vi "Auton PickUpRC.vi"() -> ()   [LabVIEW 2014]
uses:
  Robot Global Data.vi
panel:
  out "Waveform Chart":dbl(graph)
  in  "Wait Time between each step":dbl=0.5
  out "Current Step 2":string
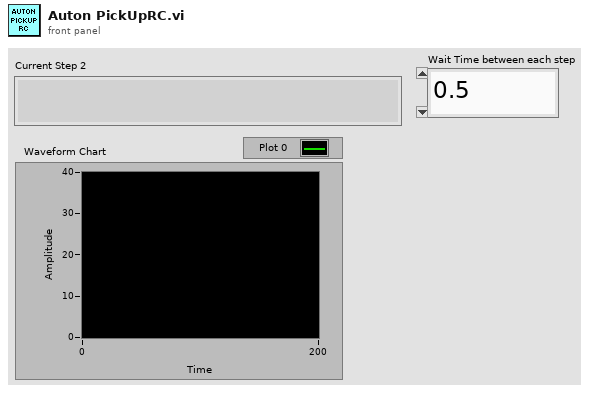
[diagram p1: front panel]
types:
  T1 = typedef "WPI_EncoderDevRef.ctl" = cluster{"DevStatus":errorcluster, "EncoderIndex":T2, "CounterIndex":T3, "DistancePerCount":dbl, "Decoding Type":T4}
  T2 = typedef "FPGA_EncoderIdx.ctl" = enum8{"Enc 0", "Enc 1", "Enc 2", "Enc 3", "Enc 4", "Enc 5", "Enc 6", "Enc 7", "Invalid"}
  T3 = typedef "FPGA_CounterCtrSystemIndex.ctl" = enum8{"Ctr 0", "Ctr 1", "Ctr 2", "Ctr 3", "Ctr 4", "Ctr 5", "Ctr 6", "Ctr 7", "Invalid"}
  T4 = typedef "WPI_EncoderType.ctl" = enum16{"1x", "2x", "4x"}
  T5 = typedef "WPI_MotorControlDeviceRef.ctl" = cluster{"DeviceStatus":errorcluster, "Type":T6, "PWM":cluster{"Controller":T7, "PWM Channel":T8, "DeadBand":T9}, "CAN":cluster{"Device Number":u8, "Control Mode":T10, "Semaphore":T11, "Max Vout":dbl, "TalonSRX Control Mode":T12}, "Invert":bool, "TransformRef":T13, "InvTransformRef":T13}
  T6 = typedef "WPI_MotorControlType.ctl" = enum16{"PWM", "CAN", "CANTalonSRX"}
  T7 = typedef "FPGA_TypedefDigitalModule.ctl" = enum16{"Controller 1"}
  T8 = typedef "FPGA_DIOPWMChannel.ctl" = enum8{"PWM 0", "PWM 1", "PWM 2", "PWM 3", "PWM 4", "PWM 5", "PWM 6", "PWM 7", "PWM 8", "PWM 9", "PWM MXP 0", "PWM MXP 1", "PWM MXP 2", "PWM MXP 3", "PWM MXP 4", "PWM MXP 5", "PWM MXP 6", "PWM MXP 7", "PWM MXP 8", "PWM MXP 9", "Invalid"}
  T9 = typedef "WPI_PWMDeadband.ctl" = cluster{"Name":string, "maxPositivePwm":i32, "minPositivePwm":i32, "centerPwm":i32, "maxNegativePwm":i32, "minNegativePwm":i32, "angularRange":u16}
  T10 = typedef "WPI_CANJaguar_ControlMode.ctl" = enum8{"Percent VBus", "Current", "Speed", "Position", "Voltage"}
  T11 = typedef "Semaphore RefNum" = refnum<k1>
  T12 = typedef "WPI_CANTalonSRX_APIControlMode.ctl" = enum8{"Percent VBus", "Speed", "Position", "Slave", "Unchanged / Invalid"}
  T13 = typedef "WPI_PWMTransform_ConPane.ctl" = refnum<vi>
  T14 = enum16{"Claw State Opening", "Claw State Opened"}
  T15 = enum16{"Claw State Open", "Claw State Closed", "Claw State Do Nothing"}
  T16 = enum16{"Elevator State Bottom", "Elevator State Clear a Tote", "Elevator State Carry a  RC", "Elevator do Nothing"}
  T17 = enum16{"Elevator Heading to Bottom", "Elevator Reached Bottom"}
  T18 = enum16{"Claw State Closing", "Claw State Closed"}
  T19 = enum16{"Claw State Closing", "Claw State Closed", "Squeeze"}
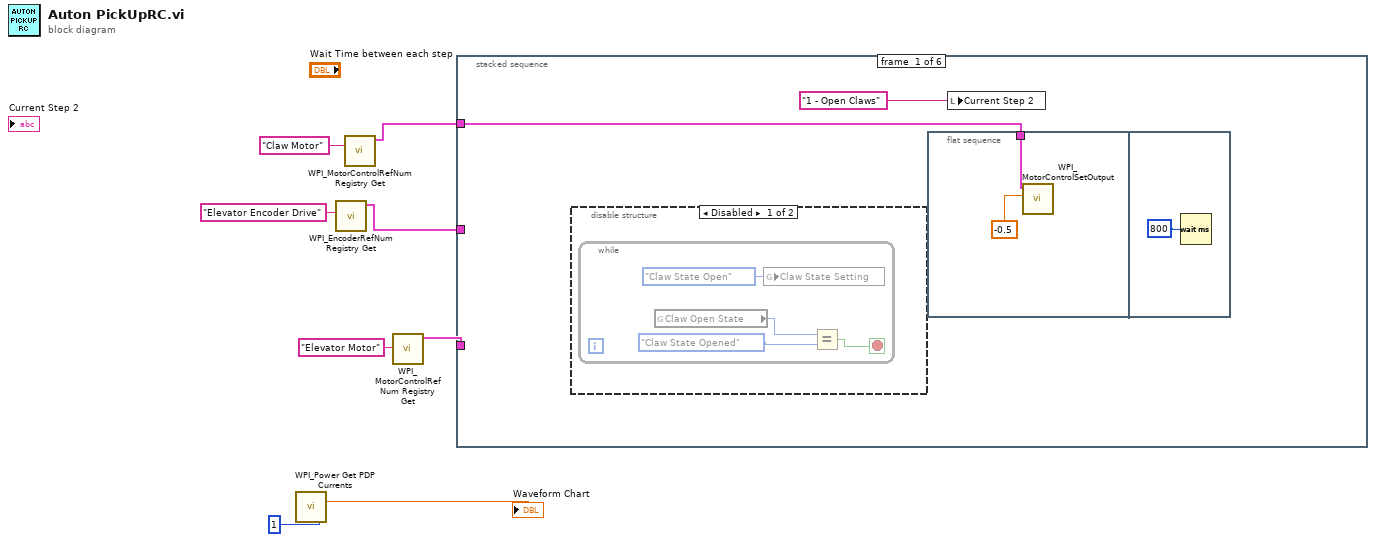
[diagram p0: block diagram]
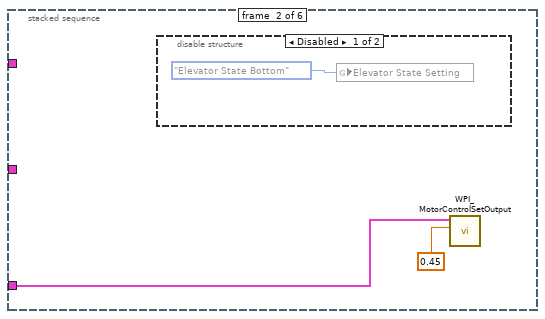
[diagram p3: hidden frame]
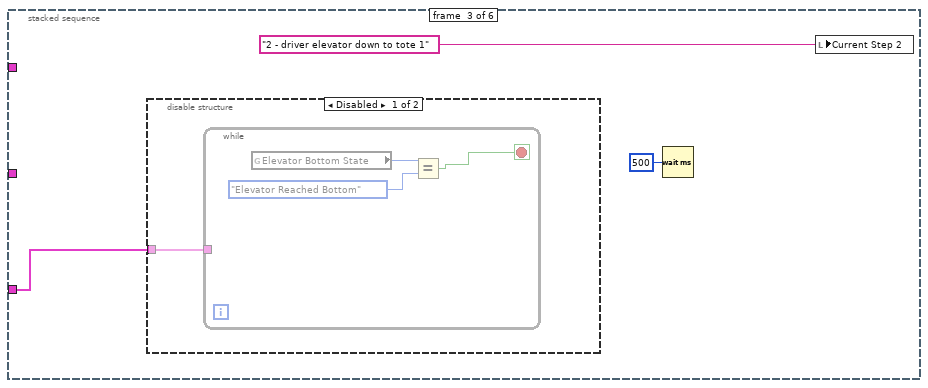
[diagram p5: hidden frame]
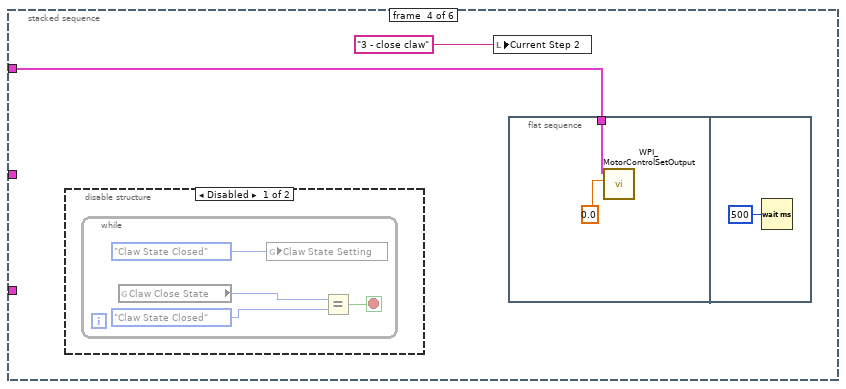
[diagram p7: hidden frame]
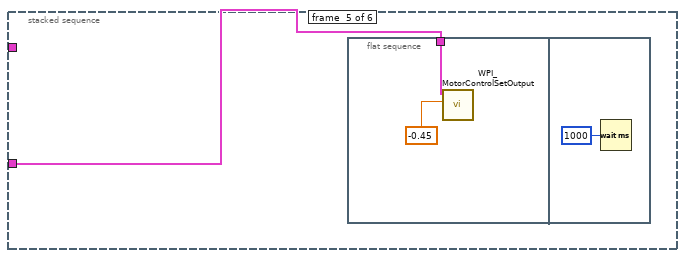
[diagram p9: hidden frame]
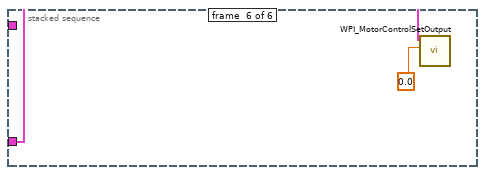
[diagram p10: hidden frame]
diagram:
  n1 = call <vilib>:"WPI_Power Get PDP Currents.vi"("PDP Channel"=1) -> ("current (A)"=→"Waveform Chart":dbl)  [unwired: 12 in, 2 out]
  n2 = call <vilib>:"WPI_EncoderRefNum Registry Get.vi"("refnum name"="Elevator Encoder Drive") -> ("EncoderDevRef"=w5:T1)  [unwired: 9 in, 1 out]
  n3 = call <vilib>:"WPI_MotorControlRefNum Registry Get.vi"("refnum name"="Claw Motor") -> ("MotorControlDevRef"=w1:T5)  [unwired: 9 in, 1 out]
  n4 = call <vilib>:"WPI_MotorControlRefNum Registry Get.vi"("refnum name"="Elevator Motor") -> ("MotorControlDevRef"=w7:T5)  [unwired: 9 in, 1 out]
  n5 = stacked-sequence {
    tunnel: w7 -> [_ w19 w22 _ w37 w42]
    tunnel: w5 -> [_ _ _ _ _ _]
    tunnel: w1 -> [w9 _ _ w28 _ _]
    frame #0 {
      n6 = disable-structure shown="Disabled" {
        frame Disabled {
          n7 = while {
            stop <- w15 stop-if-true
            n8 = global read "Robot Global Data.vi" "Claw Open State"() -> (w16:T14)
            n9 = global write "Robot Global Data.vi" "Claw State Setting"(T15."Claw State Open" ("Enum")) -> ()
            n10 = Equal?(x=w16, y=T14."Claw State Opened" ("Claw Open State")) -> (x = y?=w15:bool)
          }
        }
        frame Enabled {
        }
      }
      n11 = flat-sequence {
        tunnel: w9 -> [w11]
        frame #0 {
          n12 = call <vilib>:"WPI_MotorControlSetOutput.vi"("Output"=-0.5, "MotorControlDevRef"=w11) -> ()  [unwired: 7 in, 3 out]
        }
        frame #1 {
          n13 = Wait (ms)(milliseconds to wait=u32 800) -> ()  [unwired: 1 out]
        }
      }
      n14 = local write "Current Step 2"("1 - Open Claws" ("Current Step")) -> ()
    }
    frame #1 {
      n15 = disable-structure shown="Disabled" {
        frame Disabled {
          n16 = global write "Robot Global Data.vi" "Elevator State Setting"(T16."Elevator State Bottom" ("Elevator State Setting")) -> ()
        }
        frame Enabled {
        }
      }
      n17 = call <vilib>:"WPI_MotorControlSetOutput.vi"("Output"=0.45, "MotorControlDevRef"=w19) -> ()  [unwired: 7 in, 3 out]
    }
    frame #2 {
      n18 = disable-structure shown="Disabled" {
        disable-tunnel: w22 -> [w24 _]
        frame Disabled {
          n19 = while {
            tunnel: w24 -> [_]
            stop <- w25 stop-if-true
            n20 = global read "Robot Global Data.vi" "Elevator Bottom State"() -> (w27:T17)
            n21 = Equal?(x=w27, y=T17."Elevator Reached Bottom" ("Elevator Bottom State")) -> (x = y?=w25:bool)
          }
        }
        frame Enabled {
        }
      }
      n22 = Wait (ms)(milliseconds to wait=u32 500) -> ()  [unwired: 1 out]
      n23 = local write "Current Step 2"("2 - driver elevator down to tote 1" ("Current Step")) -> ()
    }
    frame #3 {
      n24 = disable-structure shown="Disabled" {
        frame Disabled {
          n25 = while {
            stop <- w33 stop-if-true
            n26 = global read "Robot Global Data.vi" "Claw Close State"() -> (w35:T19)
            n27 = global write "Robot Global Data.vi" "Claw State Setting"(T15."Claw State Closed" ("Enum")) -> ()
            n28 = Equal?(x=w35, y=T18."Claw State Closed" ("Claw Close State")) -> (x = y?=w33:bool)
          }
        }
        frame Enabled {
        }
      }
      n29 = local write "Current Step 2"("3 - close claw" ("Current Step")) -> ()
      n30 = flat-sequence {
        tunnel: w28 -> [w30]
        frame #0 {
          n31 = call <vilib>:"WPI_MotorControlSetOutput.vi"("Output"=0.0, "MotorControlDevRef"=w30) -> ()  [unwired: 7 in, 3 out]
        }
        frame #1 {
          n32 = Wait (ms)(milliseconds to wait=u32 500) -> ()  [unwired: 1 out]
        }
      }
    }
    frame #4 {
      n33 = flat-sequence {
        tunnel: w37 -> [w38]
        frame #0 {
          n34 = call <vilib>:"WPI_MotorControlSetOutput.vi"("Output"=-0.45, "MotorControlDevRef"=w38) -> ()  [unwired: 7 in, 3 out]
        }
        frame #1 {
          n35 = Wait (ms)(milliseconds to wait=u32 1000) -> ()  [unwired: 1 out]
        }
      }
    }
    frame #5 {
      n36 = call <vilib>:"WPI_MotorControlSetOutput.vi"("Output"=0.0, "MotorControlDevRef"=w42) -> ()  [unwired: 7 in, 3 out]
    }
  }
